vi "HXG2_HeatLoadAir.vi"(1 "Pbaro (psia)":dbl, 2 "Mdot Air (lbm/hr)":dbl, 7 "%RH UUT":dbl, 9 "dP UUT (inWC)":dbl, 11 "error in (no error)":errorcluster, 12 "Air In Avg (°F)":dbl, 13 "Air Out Avg (°F)":dbl) -> (4 "Q air (BTU/hr)":dbl, 6 "Qair (W)":dbl, 8 "CFM HX":dbl, 10 "Moist Air Cp (BTU/lb)":dbl, 14 "Moist Air Density (lbm/ft³)":dbl, 15 "error out":errorcluster)   [LabVIEW 2012]
doc: "This VI will comlplete psychrometric calculations and output density of air and complete the calculation to figure out the heat load on the air side and finalizes with the conversion from SCFM to ACFM. The ACFM calculation is documented at the bottom of the block diagram."
panel:
  out "Qair Std":dbl
  out "Cp Wtr (BTU/lbm R)":dbl
  out "Cp Dry Air (BTU/lbm R)":dbl
  out "Eqn used Pws":dbl
  out "v (lbs/lbs dry air)":sgl
  out "Pw":sgl
  out "T R":sgl
  out "Patm":sgl
  out "Pws":sgl
  out "W HX in":dbl
  out "Inlet Enthalpy (BTU/lb)":sgl
  out "Outlet Enthalpy (BTU/lb)":sgl
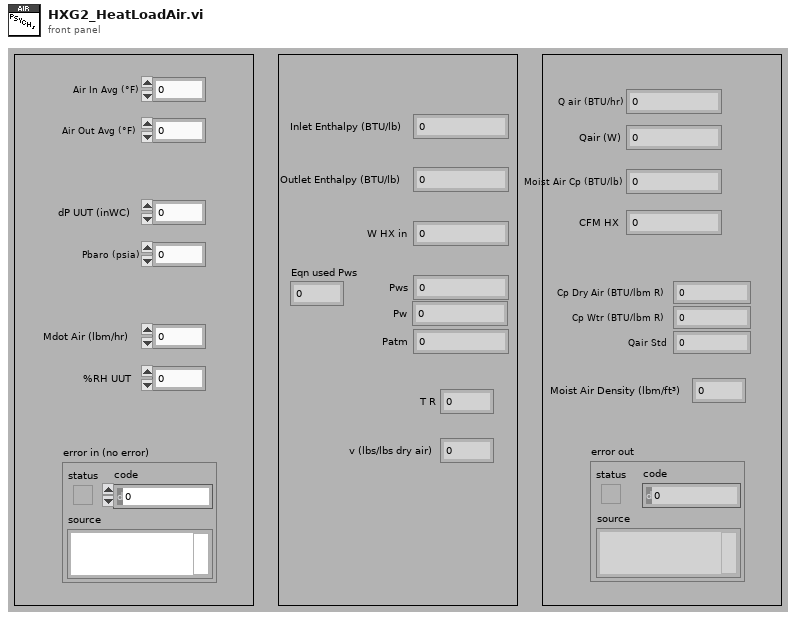
[diagram p1: front panel]
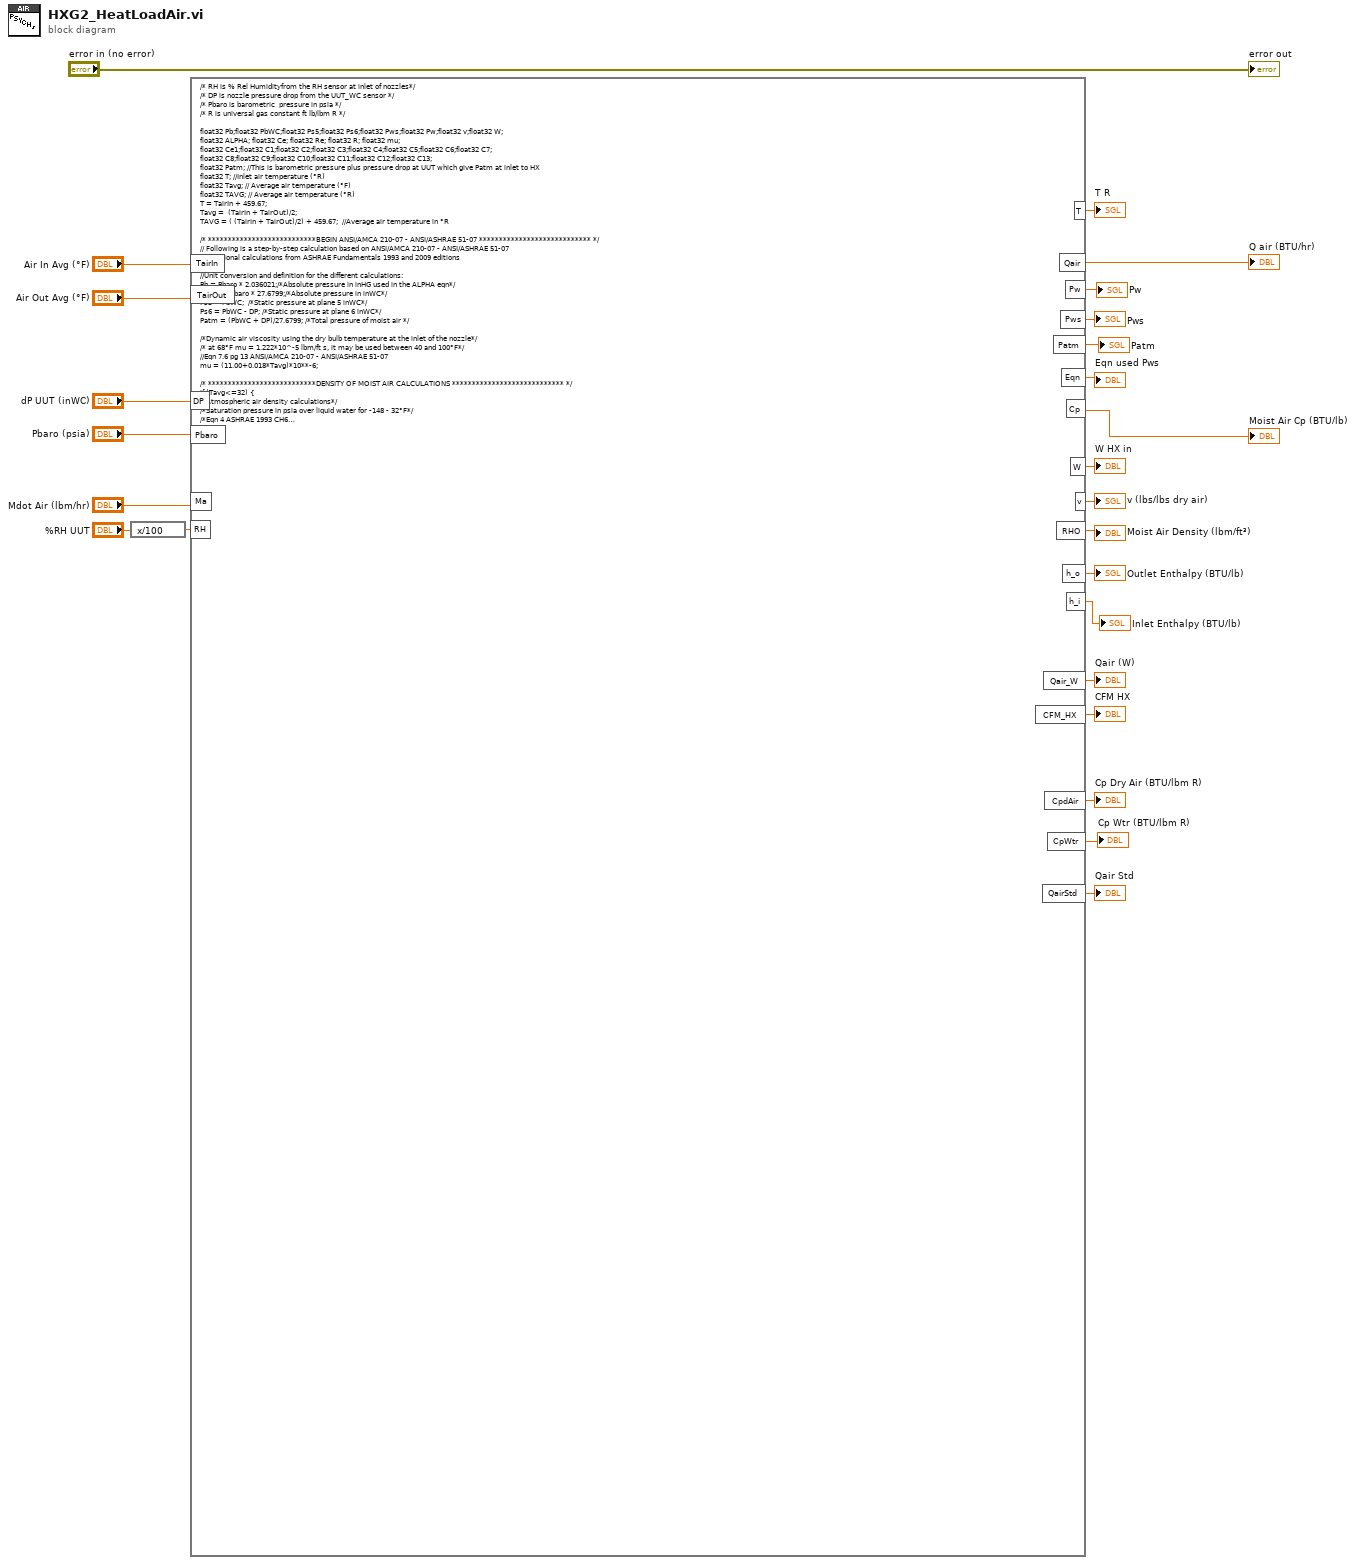
[diagram p0: block diagram]
diagram:
  n1 = expression code="x/100"("%RH UUT") -> (w9:dbl)
  n2 = formula code="/* RH is % Rel Humidityfrom the RH sensor at inlet of nozzles*/\n/* DP is nozzle pressure drop from the UUT_WC sensor */\n/* Pbaro is barometric  pressure in psia */ \n/* R is universal gas constant ft lb/lbm R */\n\nfloat32 Pb;float32 PbWC;float32 Ps5;float32 Ps6;float32 Pws;float32 Pw;float32 v;float32 W;\nfloat32 ALPHA; float32 Ce; float32 Re; float32 R; float32 mu;\nfloat32 Ce1;float32 C1;float32 C2;float32 C3;float32 C4;float32 C5;float32 C6;float32 C7;\nfloat32 C8;float32 C9;float32 C10;float32 C11;float32 C12;float32 C13;\nfloat32 Patm; //This is barometric pressure plus pressure drop at UUT which give Patm at inlet to HX\nfloat32 T; //Inlet air temperature (°R)\nfloat32 Tavg; // Average air temperature (°F)\nfloat32 TAVG; // Average air temperature (°R)\nT = TairIn + 459.67;\nTavg =  (TairIn + TairOut)/2;\nTAVG = ( (TairIn + TairOut)/2) + 459.67;  //Average air temperature in °R\n\n/* ***************************BEGIN ANSI/AMCA 210-07 - ANSI/ASHRAE 51-07 **************************** */\n// Following is a step-by-step calculation based on ANSI/AMCA 210-07 - ANSI/ASHRAE 51-07\n// Additional calculations from ASHRAE Fundamentals 1993 and 2009 editions\n\n//Unit conversion and definition for the different calculations:\nPb = Pbaro * 2.036021;/*Absolute pressure in inHG used in the ALPHA eqn*/\nPbWC = Pbaro * 27.6799;/*Absolute pressure in inWC*/\nPs5 = PbWC;  /*Static pressure at plane 5 inWC*/\nPs6 = PbWC - DP; /*Static pressure at plane 6 inWC*/\nPatm = (PbWC + DP)/27.6799; /*Total pressure of moist air */\n\n/*Dynamic air viscosity using the dry bulb temperature at the inlet of the nozzle*/\n/* at 68°F mu = 1.222*10^-5 lbm/ft s, it may be used between 40 and 100°F*/\n//Eqn 7.6 pg 13 ANSI/AMCA 210-07 - ANSI/ASHRAE 51-07\nmu = (11.00+0.018*Tavg)*10**-6;\n\n/* ***************************DENSITY OF MOIST AIR CALCULATIONS **************************** */\nif (Tavg<=32) {\n/*Atmospheric air density calculations*/\n/*Saturation pressure in psia over liquid water for -148 - 32°F*/\n/*Eqn 4 ASHRAE 1993 CH6*/\nC1 = -1.0214165*10**4;\nC2 = -4.8932428*10**0;\nC3 = -5.3765794*10**-3;\nC4 = 1.9202377*10**-7;\nC5 = 3.5575832*10**-10;\nC6 = -9.0344688*10**-14;\nC7 = 4.1635019;\nPws = exp(C1/T + C2 + C3*T + C4*T**2 + C5*T**3 + C6*T**4 + C7*ln(T)); /*psia*/\nEqn = 1;\n}\nelse{\n/*Atmospheric air density calculations*/\n/*Saturation pressure in psia over liquid water for 32-392°F*/\n/*Eqn 4 ASHRAE 1993 CH6*/\nC8 = -1.0440397*10**4;\nC9 = -1.1294650*10**1;\nC10 = -2.7022355*10**-2;\nC11= 1.2890360*10**-5;\nC12 = -2.4780681*10**-9;\nC13 = 6.5459673;\nPws = exp(C8/T + C9 + C10*T + C11*T**2 + C12*T**3 +C13*ln(T)); /*psia*/\nEqn = 2;\n}\n/*Partial pressure of water vapor (Pw=Pe)*/\n/*Eqn 22 ASHRAE 1993 CH6*/\nPw = RH*Pws; /*psia*/\n\n/*Humidity ratio W*/\n/*Total pressure of moist air in psi is Patm*/\n/*Eqn 23 ASHRAE 2009 CH1*/\nW = 0.621945*(Pw/(Patm-Pw));\n\n/*Specific volume of moist air mixture v*/\n/*Eqn 28 ASHRAE 2009 CH1*/\nv = 0.370486*T*(1+1.607858*W)/Patm; /*cft/lbs of dry air*/\n\n/*Density of Moist Air*/\n/*Eqn 11 ASHRAE 1993 CH6*/\nRHO = (1/v)*(1+W);\n/* ***********************END DENSITY OF MOIST AIR CALCULATIONS **************************** */\nh_i = 0.240*TairIn+ W*(1061+0.444*TairIn);\nh_o = 0.240*TairOut+ W*(1061+0.444*TairOut);\n/* ***********************END OF MOIST AIR CALCULATIONS **************************** */\n\nCFM_HX = Ma / RHO*(1/60);\n\n/* ***********************Calculate Cp at Average air temp **************************** */\n\n/*Specific heat of dry air*/\nCpdAir = 0.246584621 + -0.0000272742883681093*TAVG  + 2.97554208740569E-08*TAVG**2; //BTU/lbm R\n/*Specific heat of water*/\nCpWtr= -0.000000000000432128*(TAVG**5) + 0.00000000131349*(TAVG**4) - 0.00000159567*(TAVG**3) + 0.000969041*(TAVG**2) - 0.294304*(TAVG) + 36.7663;\n\nCp = CpdAir * (1-W) + W*CpWtr; //Cp of moist air\n\n//Heat load Air side\nQair = Ma*Cp*(TairOut-TairIn);\nQair_W = Qair / 3.415179; //Qair in Watts"("TairIn"="Air In Avg (°F)", "Pbaro"="Pbaro (psia)", "TairOut"="Air Out Avg (°F)", "DP"="dP UUT (inWC)", "Ma"="Mdot Air (lbm/hr)", "RH"=w9) -> ("Qair"=→"Q air (BTU/hr)":dbl, "Cp"=→"Moist Air Cp (BTU/lb)":dbl, "h_o"=→"Outlet Enthalpy (BTU/lb)":dbl, "h_i"=→"Inlet Enthalpy (BTU/lb)":dbl, "W"=→"W HX in":sgl, "Pws"=→"Pws":sgl, "Patm"=→"Patm":sgl, "T"=→"T R":sgl, "Pw"=→"Pw":sgl, "v"=→"v (lbs/lbs dry air)":sgl, "RHO"=→"Moist Air Density (lbm/ft³)":dbl, "Eqn"=→"Eqn used Pws":dbl, "Qair_W"=→"Qair (W)":dbl, "CFM_HX"=→"CFM HX":dbl, "CpdAir"=→"Cp Dry Air (BTU/lbm R)":dbl, "CpWtr"=→"Cp Wtr (BTU/lbm R)":dbl, "QairStd"=→"Qair Std":dbl)
  "error out" <- "error in (no error)"
